vi "Start Dependency.vi"(7 "Owner":refnum<class "SMO.lvclass">, 8 "error in (no error)":errorcluster, 11 "Dependency in":refnum<class "Dependency.lvclass">) -> (0 "error out":errorcluster, 3 "Dependency out":refnum<class "Dependency.lvclass">)   [LabVIEW 2013, in "Dependency.lvclass"]
uses:
  Dependency.lvclass
  SMO/SMO.lvclass
  Dependency.lvclass/Dependency.ctl
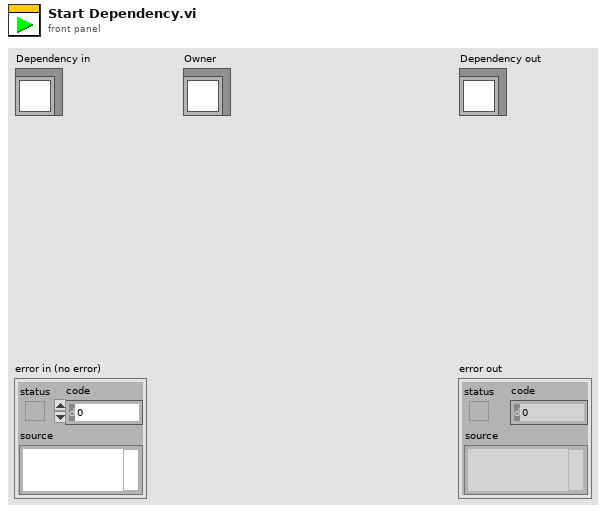
[diagram p1: front panel]
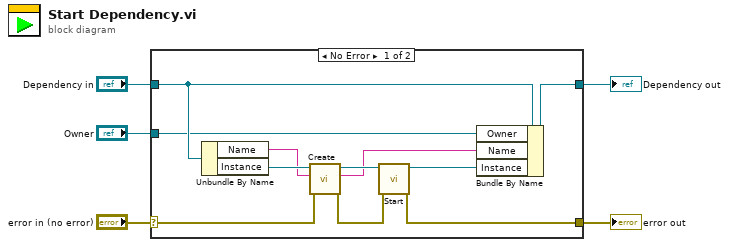
[diagram p0: block diagram]
diagram:
  n1 = case shown="No Error" "error in (no error)" {
    selector: "error in (no error)" -> [w11 w18]
    tunnel: [w10 w18] -> w4
    tunnel: [w9 w17] -> w2
    tunnel: "Dependency in" -> [w16 w17]
    tunnel: "Owner" -> [w7 _]
    frame No Error {
      n2 = Unbundle By Name(w16) -> ("Name"=w6:string, "Instance"=w13:refnum<class "SMO.lvclass">)
      n3 = call "Create.vi"("error in (no error)"=w11, "Subsystem Name (optional)"=w6, "SMO"=w13) -> ("error out"=w14:errorcluster, "SMO name"=w8:string, "SMO out"=w15:refnum<class "SMO.lvclass">)  [unwired: 6 in]
      n4 = call "Start.vi"("error in (no error)"=w14, "SMO"=w15) -> ("error out"=w10:errorcluster, "SMO out"=w12:refnum<class "SMO.lvclass">)  [unwired: 8 in]
      n5 = Bundle By Name(cluster=w16, "Owner"=w7, "Name"=w8, "Instance"=w12) -> (w9:refnum<class "Dependency.lvclass">)
    }
    frame Error {
    }
  }
  "error out" <- w4
  "Dependency out" <- w2
